vi "In-Place Debug.vi"(2 "Input":bool, 3 "Action":T1) -> (0 "Output":bool)   [LabVIEW 2013]
uses:
  src/Functional Globals/Action.ctl
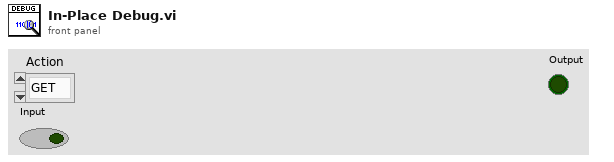
[diagram p1: front panel]
types:
  T1 = typedef "Action.ctl" = enum16{"GET", "PUT", "DELETE"}
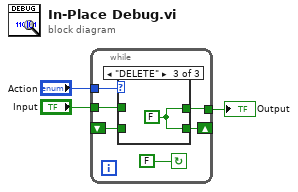
[diagram p0: block diagram]
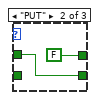
[diagram p3: hidden frame]
diagram:
  n1 = while {
    shift-right: [w7] -> _
    shift-left: _ -> [w8]
    tunnel: "Action" -> [w6]
    tunnel: "Input" -> [w5]
    tunnel: [w4] -> w1
    stop <- FALSE continue-if-true
    n2 = case shown="\"DELETE\"" w6 {
      tunnel: w8 -> [w10 _ _]
      tunnel: [w10 w12 w13] -> w7
      tunnel: w5 -> [_ w12 _]
      tunnel: [w10 FALSE ("Input") w13] -> w4
      frame "GET", Default {
      }
      frame "PUT" {
      }
      frame "DELETE" {
        w13 = FALSE ("Input")
      }
    }
  }
  "Output" <- w1
